vi "05. Native MQTT Service Provider.vi"() -> ()   [LabVIEW 2019]
uses:
  Actor/Request -- cluster.ctl
  <vilib>/LabVIEW Open Source Project/MQTT Control Packets/Control Packets/ControlPacket/ControlPacket.lvclass/ControlPacket.ctl
  d83398bf-d288-4447-9c56-1851baa950d7.vi
  <vilib>/LabVIEW Open Source Project/MQTT Control Packets/Control Packets/PUBLISH/PUBLISH.lvclass
  C:/Program Files (x86)/National Instruments/LabVIEW 2019/vi.lib/LabVIEW Open Source Project/MQTT Control Packets/Control Packets/ControlPacket/ControlPacket.lvclass
  <vilib>/JDP Science/JSONtext/JSON text to Variant.vi
  <vilib>/JDP Science/JSONtext/LVClass Serializer/JSONtext LVClass Serializer.lvclass
  <vilib>/LabVIEW Open Source Project/MQTT Control Packets/Control Packets/ControlPacket/ControlPacket.lvclass
  <vilib>/JDP Science/JSONtext/JSONtext.lvlib
panel:
  out "<JSON>":string caption="<JSON>Request"
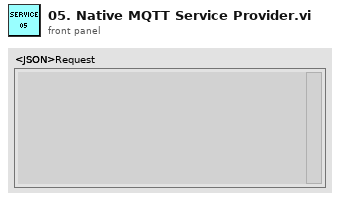
[diagram p1: front panel]
types:
  T1 = typedef "Actor Private Data.ctl" = cluster{"Client":refnum<class "Client.lvclass">, "QualifiedName":string, "EventReg":refnum<event-registration>, "Private Events":T2}
  T2 = typedef "Actor Private Events -- cluster.ctl" = cluster{"Stop":refnum<user-event>, "Subscribe":refnum<user-event>, "Unsubscribe":refnum<user-event>, "publish":refnum<user-event>}
  T3 = typedef "Request -- cluster.ctl" = cluster{"method":string, "<JSON>params":string, "id":string, "reply-topic":string}
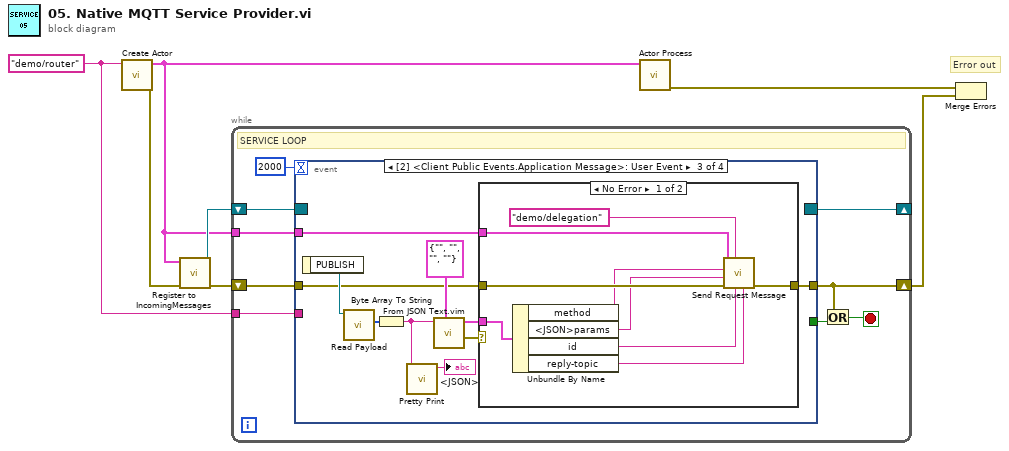
[diagram p0: block diagram]
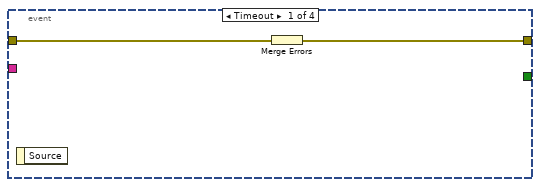
[diagram p2: hidden frame]
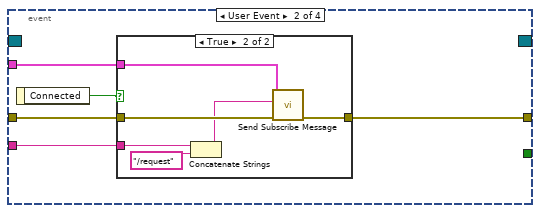
[diagram p3: hidden frame]
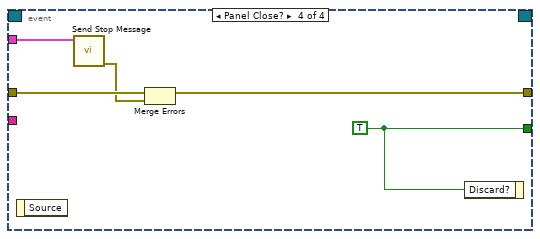
[diagram p6: hidden frame]
diagram:
  w2 = "demo/router" ("QualifiedName")
  # "Error out"
  n1 = call "Create Actor.vi"("QualifiedName"=w2) -> ("error out"=w6:errorcluster, "Actor Class"=w4:T1)  [unwired: 9 in]
  n2 = call "Register to IncomingMessages.vi"("error in"=w6, "Actor Class"=w4) -> ("error out"=w3:errorcluster, "Incoming Messages"=w5:refnum<event-registration>)  [unwired: 8 in]
  n3 = while {
    tunnel: w4 -> [w14]
    shift-right: [w11] -> _
    shift-left: w5 -> [w12]
    shift-right: [w9] -> w1
    shift-left: w3 -> [w10]
    tunnel: w2 -> [w8]
    stop <- w15 stop-if-true
    # "SERVICE LOOP"
    n4 = event shown="[2] <Client Public Events.Application Message>: User Event" {
      selector: w12 -> [_ _ _ _]
      dyn-events: [_ _ _ _] -> w11
      timeout: 2000 -> [_ _ _ _]
      tunnel: [_ _ _ w55] -> w16
      tunnel: w14 -> [_ w21 w35 w54]
      tunnel: [w17 w22 w33 w51] -> w9
      tunnel: w10 -> [w18 w23 w34 w53]
      tunnel: w8 -> [_ w19 _ _]
      event Timeout {
        n5 = event-data() -> ()  [unwired: 1 in, 1 out]
        n6 = Merge Errors(w18) -> (w17:errorcluster)
      }
      event User Event {
        n7 = event-data() -> ("Connected"=w20:bool)  [unwired: 1 in]
        n8 = case shown="True" w20 {
          tunnel: w23 -> [w24 w30]
          tunnel: [w24 w29] -> w22
          tunnel: w21 -> [_ w28]
          tunnel: w19 -> [_ w27]
          frame False {
          }
          frame True {
            n9 = Concatenate Strings(w27, "/request" ("QualifiedName")) -> (w25:string)
            n10 = call "Send Subscribe Message.vi"("error in"=w30, "Topic"=w25, "Actor Class"=w28) -> ("error out"=w29:errorcluster)  [unwired: 8 in]
          }
        }
      }
      event User Event {
        n11 = event-data() -> ("PUBLISH"=w40:refnum<class "PUBLISH.lvclass">)  [unwired: 1 in]
        n12 = call <vilib>:"Read Payload.vi"("ControlPacket in"=w40) -> ("Payload"=w39:u8[])  [unwired: 9 in, 1 out]
        n13 = Byte Array To String(unsigned byte array=w39) -> (string=w32:string)
        n14 = call <vilib>:"Pretty Print.vi"("JSON"=w32) -> ("<JSON>"=→"<JSON>":string)  [unwired: 8 in, 2 out]
        n15 = call "From JSON Text.vim"("Data Type and Default Value"=T3 {"method"="", "<JSON>params"="", "id"="", "reply-topic"=""} ("request"), "JSON"=w32) -> ("error out"=w37:errorcluster, "Data out"=w36:T3)  [unwired: 8 in]
        n16 = case shown="No Error" w37 {
          tunnel: w36 -> [w43 _]
          tunnel: w35 -> [w47 _]
          tunnel: w34 -> [w49 w50]
          tunnel: [w48 w50] -> w33
          frame No Error {
            n17 = Unbundle By Name(w43) -> ("method"=w45:string, "<JSON>params"=w44:string, "id"=w42:string, "reply-topic"=w41:string)
            n18 = call "Send Request Message.vi"("reply-topic"=w41, "id"=w42, "Qualified Name"="demo/delegation" ("QualifiedName"), "error in"=w49, "<JSON>params"=w44, "method"=w45, "Actor Class"=w47) -> ("error out"=w48:errorcluster)  [unwired: 2 in, 2 out]
          }
          frame Error {
            # "Invalid request payload"
          }
        }
      }
      event Panel Close? {
        w55 = TRUE ("Discard?")
        n19 = event-data() -> ()  [unwired: 1 in, 1 out]
        n20 = call "Send Stop Message.vi"("Actor Class"=w54) -> ("error out"=w52:errorcluster)  [unwired: 10 in]
        n21 = Merge Errors(w53, w52) -> (w51:errorcluster)
        n22 = event-data("Discard?"=w55) -> ()  [unwired: 1 in, 1 out]
      }
    }
    n23 = Or(x=w9, y=w16) -> (x .or. y?=w15:bool)
  }
  n24 = call "Actor Process.vi"("Actor Class"=w4) -> ("error out"=w7:errorcluster)  [unwired: 10 in]
  n25 = Merge Errors(w7, w1) -> ()  [unwired: 1 out]
